vi "Untitled 2.vi"() -> ()   [LabVIEW 2011]
panel:
  out "Waveform Chart":dbl(graph)
  in  "stop":bool
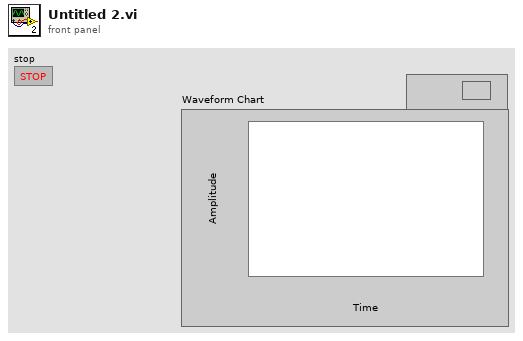
[diagram p1: front panel]
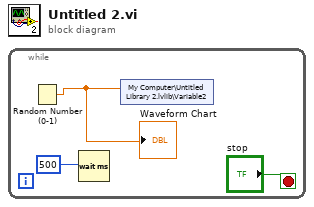
[diagram p0: block diagram]
diagram:
  n1 = while {
    stop <- "stop" stop-if-true
    n2 = Random Number (0-1)() -> (number: 0 to 1=w1:dbl)
    "Waveform Chart" <- w1
    n3 = Wait (ms)(milliseconds to wait=u32 500 ("millisecond timer value")) -> ()  [unwired: 1 out]
    n4 = shared-variable "My Computer\\Untitled Library 2.lvlib\\Variable2"(w1) -> ()  [unwired: 1 in, 1 out]
  }
